vi "Pulse Generator.vi"(8 "error in (no error)":errorcluster, 11 "Pulse Generator in":refnum<class "Pulse Generator.lvclass">) -> (0 "error out":errorcluster, 3 "Pulse Generator out":refnum<class "Pulse Generator.lvclass">)   [LabVIEW 2012, in "Pulse Generator.lvclass"]
uses:
  Pulse Generator.lvclass
  Global/GPIB Numbers.vi
panel:
  out "Status":string
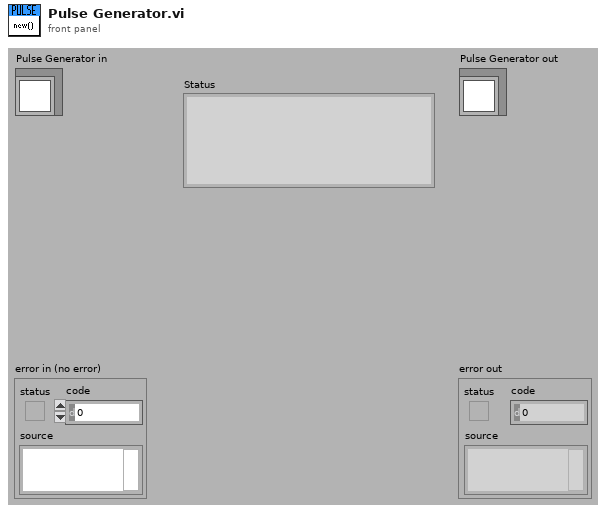
[diagram p1: front panel]
types:
  T1 = typedef "GPIB Type Def.ctl" = cluster{"Name":string, "bus":dbl, "GPIB":dbl, "GPIB as string":string, "byte":i32, "VISA Resource Name":refnum<visa-resource-name>}
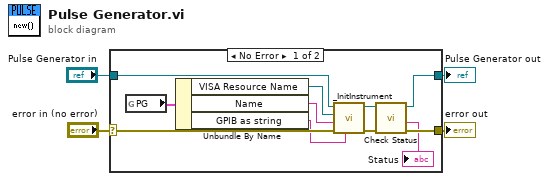
[diagram p0: block diagram]
diagram:
  n1 = case shown="No Error" "error in (no error)" {
    selector: "error in (no error)" -> [w14 w17]
    tunnel: [w6 w17] -> w3
    tunnel: [w8 w16] -> w1
    tunnel: "Pulse Generator in" -> [w15 w16]
    frame No Error {
      n2 = global read "GPIB Numbers.vi" "PG"() -> (w13:T1)
      n3 = Unbundle By Name(w13) -> ("VISA Resource Name"=w12:refnum<visa-resource-name>, "Name"=w11:string, "GPIB as string"=w10:string)
      n4 = call-dynamic "_InitInstrument.vi"("GPIB as string"=w10, "error in (no error)"=w14, "Name"=w11, "VISA Resource Name"=w12, "Instrument in"=w15) -> ("error out"=w7:errorcluster, "Instrument out"=w9:refnum<class "Pulse Generator.lvclass">)  [unwired: 5 in]
      n5 = call-dynamic "Check Status.vi"("error in (no error)"=w7, "Pulse Generator in"=w9) -> ("error out"=w6:errorcluster, "Status"=→"Status":string, "Pulse Generator out"=w8:refnum<class "Pulse Generator.lvclass">)  [unwired: 7 out]
    }
    frame Error {
    }
  }
  "error out" <- w3
  "Pulse Generator out" <- w1
